vi "Receive High Speed Data Queue.vi"(8 "error in (no error)":errorcluster, 9 "timeout in ms (-1)":i32=-1, 11 "Message Enqueuer":refnum<class "Message Enqueuer.lvclass">) -> (0 "error out":errorcluster, 2 "High Speed Data Queue":refnum<queue>, 3 "Message Enqueuer out":refnum<class "Message Enqueuer.lvclass">)   [LabVIEW 2024]
uses:
  <vilib>/ActorFramework/Message Enqueuer/Message Enqueuer.lvclass
  Analog Reader Messages/Get High Speed Data Queue Msg/Get High Speed Data Queue Msg.lvclass/Get High Speed Data Queue Msg.ctl
  <vilib>/ActorFramework/Message Enqueuer/Message Enqueuer.lvclass/Message Enqueuer.ctl
  <vilib>/ActorFramework/Message Enqueuer/Enqueue.vi
  Analog Reader Messages/Get High Speed Data Queue Msg/Get High Speed Data Queue Msg.lvclass
  <vilib>/ActorFramework/Message Priority Queue/Priority Enqueue.vi
  Analog Reader.lvclass/Analog Reader.ctl
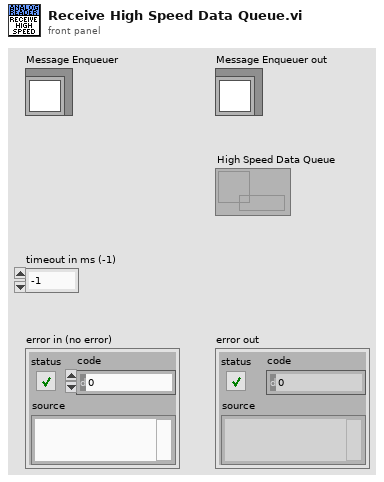
[diagram p1: front panel]
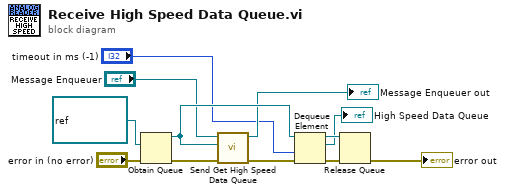
[diagram p0: block diagram]
diagram:
  n1 = Obtain Queue(element data type=refnum<queue> refnum ("High Speed Data"), error in (no error)="error in (no error)") -> (queue out=w10:refnum<queue>, error out=w11:errorcluster)  [unwired: 3 in, 1 out]
  n2 = call "Send Get High Speed Data Queue.vi"("error in (no error)"=w11, "Queue of Queue"=w10, "Message Enqueuer"="Message Enqueuer") -> ("error out"=w9:errorcluster, "Message Enqueuer out"=→"Message Enqueuer out":refnum<class "Message Enqueuer.lvclass">)  [unwired: 7 in]
  n3 = Dequeue Element(queue=w10, timeout in ms (-1)="timeout in ms (-1)", error in (no error)=w9) -> (queue out=w8:refnum<queue>, element=→"High Speed Data Queue":refnum<queue>, error out=w7:errorcluster)  [unwired: 1 out]
  n4 = Release Queue(queue=w8, error in (no error)=w7) -> (error out=→"error out":errorcluster)  [unwired: 1 in, 2 out]
